vi "RIMAS Detector Init.vi"(8 "Error In":errorcluster, 11 "Detector Config":T1={"Detector"=0, "Offsets"=[[0, 0, 0, 0, 0, 0, 0, 0, 0, 0, 0, 0, 0, 0, 0, 0, 0, 0, 0, 0, 0, 0, 0, 0, 0, 0, 0, 0, 0, 0, 0, 0]], "Detector Computer"={"Machine"="192.168.121.11", "Password"="", "FITS File Path"="", "Port"=44444, "Header Path"="", "Name"=""}, "FITS hdr template0"=path "", "FITS hdr template1"=path "", "FITS Data File Path"=path "", "FITS Detector Settings"={"Exp Time Short"=0.0, "# of Frames"=0.0, "Exp Time Long"=0.0, "# of Groups"=0.0, "Object Name"="", "Object"="", "Obs Type"="", "Image Type"="", "Observer"="", "Observer Affiliation"=""}, "Sim Folder"=path "", "Integration Mode"=enum."SSR", "Integration Time"=0.0, "Frame Int Time"=0.0} {"Offsets" format="%04x"; "Detector" items=["0", "1", "2"]}) -> (0 "Error Out":errorcluster, 2 "Log Message":string, 3 "Detector Ref":refnum<k5>)   [LabVIEW 2024]
uses:
  RIMAS Detector Config.ctl
  RIMAS Detector Server Config.ctl
  RIMAS Observation Config.ctl
  Detector enum Detector Integration Mode.ctl
panel:
  # "sec"
  # "sec"
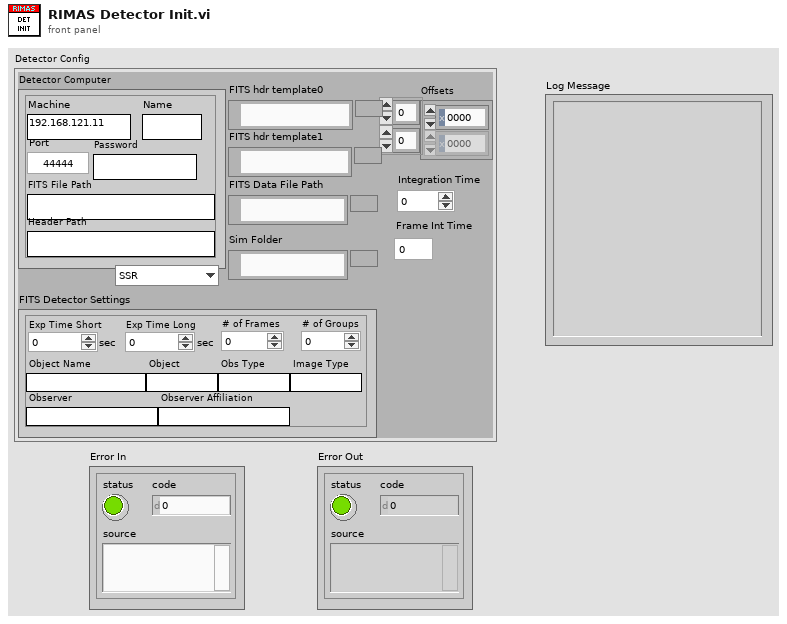
[diagram p1: front panel]
types:
  T1 = typedef "RIMAS Detector Config.ctl" = cluster{"Detector":u16, "Offsets":u16[][], "Detector Computer":T2, "FITS hdr template0":path, "FITS hdr template1":path, "FITS Data File Path":path, "FITS Detector Settings":T3, "Sim Folder":path, "Integration Mode":T4, "Integration Time":dbl, "Frame Int Time":dbl}
  T2 = typedef "RIMAS Detector Server Config.ctl" = cluster{"Machine":string, "Password":string, "FITS File Path":string, "Port":u16, "Header Path":string, "Name":string}
  T3 = typedef "RIMAS Observation Config.ctl" = cluster{"Exp Time Short":dbl, "# of Frames":dbl, "Exp Time Long":dbl, "# of Groups":dbl, "Object Name":string, "Object":string, "Obs Type":string, "Image Type":string, "Observer":string, "Observer Affiliation":string}
  T4 = typedef "Detector enum Detector Integration Mode.ctl" = enum16{"SSR", "CDS", "MEAN", "MEDIAN", "MODE", "MIIN", "MAX"}
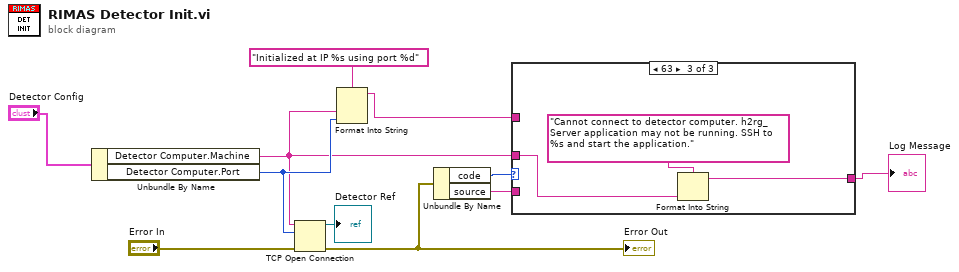
[diagram p0: block diagram]
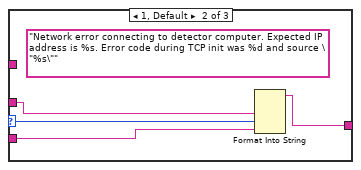
[diagram p3: hidden frame]
diagram:
  n1 = Unbundle By Name("Detector Config") -> ("Detector Computer.Machine"=w4:string, "Detector Computer.Port"=w7:u16)
  n2 = TCP Open Connection(address=w4, remote port or service name=w7, error in (no error)="Error In") -> (connection ID=→"Detector Ref":refnum<k5>, error out=w6:errorcluster)  [unwired: 2 in]
  "Error Out" <- w6
  n3 = Format Into String(format string="Initialized at IP %s using port %d", w4, w7) -> (resulting string=w2:string)  [unwired: 2 in, 1 out]
  n4 = Unbundle By Name(w6) -> ("code"=w5:i32, "source"=w1:string)
  n5 = case shown="63" w5 {
    selector: w5 -> [_ w15 _]
    tunnel: w4 -> [_ w16 w18]
    tunnel: [w12 w13 w17] -> w3
    tunnel: w2 -> [w12 _ _]
    tunnel: w1 -> [_ w14 _]
    frame 0 {
    }
    frame 1, Default {
      (unwired) "Network error connecting to detector computer. Expected IP address is %s. Error code during TCP init was %d and source \"%s\"" ("format string")
      n6 = Format Into String(w16, w15, w14) -> (resulting string=w13:string)  [unwired: 3 in, 1 out]
    }
    frame 63 {
      n7 = Format Into String(format string="Cannot connect to detector computer. h2rg_Server application may not be running. SSH to %s and start the application.", w18) -> (resulting string=w17:string)  [unwired: 2 in, 1 out]
    }
  }
  "Log Message" <- w3
